vi "Rx Streaming (Four Channels) (Host)(old).vi"() -> ()   [LabVIEW 2021]
doc: "This template is for the Simple NI-USRP Streaming design, a design that shows the basics of streaming data from an NI 294x/295x device. Refer to the block diagram for more information about how to use this template."
uses:
  SubVIs/Start Trigger.ctl
  <vilib>/userdefined/Silver/nirio_resource_slv.ctl
  <vilib>/Utility/error.llb/DialogType.ctl
  <vilib>/measure/maspectr.llb/FFT Power Spectrum and PSD for 1 Chan (CDB).vi
  <vilib>/measure/NI_MAPro.lvlib
panel:
  in  "rx config":T2={"transfer mode"=enum."Finite", "sample rate"=10000000.0, "number of samples"=8192, "start trigger"=enum."Immediate", "daughterboard 0 config"={"rf enable 0"=TRUE, "rf config 0"={"antenna"="RX1", "frequency"=5000000000.0, "gain"=40.0}, "rf enable 1"=TRUE, "rf config 1"={"antenna"="RX2", "frequency"=5000000000.0, "gain"=40.0}, "lo configuration"=enum."Shared"}, "daughterboard 1 config"={"rf enable 2"=TRUE, "rf config 2"={"antenna"="RX1", "frequency"=5000000000.0, "gain"=40.0}, "rf enable 3"=TRUE, "rf config 3"={"antenna"="RX2", "frequency"=5000000000.0, "gain"=40.0}, "lo configuration"=enum."Shared"}} {"daughterboard 1 config"."rf config 3"."gain" format="%#.1f"; "daughterboard 1 config"."rf config 3"."frequency" format="%#.3pHz"; "daughterboard 1 config"."rf config 2"."gain" format="%#.1f"; "daughterboard 1 config"."rf config 2"."frequency" format="%#.3pHz"; "daughterboard 0 config"."rf config 1"."gain" format="%#.1f"; "daughterboard 0 config"."rf config 1"."frequency" format="%#.3pHz"; "daughterboard 0 config"."rf config 0"."gain" format="%#.1f"; "daughterboard 0 config"."rf config 0"."frequency" format="%#.3pHz"; "sample rate" format="%#.3pS/s"}
  out "acquiring":bool caption="Acquiring"
  in  "USRP RIO device":T3="RIO0" caption="USRP RIO Device"
  in  "reference frequency source":string(combo)="Internal" caption="Reference Frequency Source"
  in  "indicator tab":T4(tab)
  out "power spectrum":cluster{"f0":dbl, "df":dbl, "magnitude":dbl[]}[](graph) caption="Power Spectrum"
  out "iq data":waveform(dbl)[](graph) caption="I & Q Data"
  out "rx.coerced config":T5 caption="Coerced Configurations" {"channel 3"."sample rate" format="%#.3pS/s"; "channel 3"."gain" format="%#_1f"; "channel 3"."if2 lo" format="%#.3pHz"; "channel 3"."if1 lo" format="%#.3pHz"; "channel 3"."frequency" format="%#.3pHz"; "channel 2"."sample rate" format="%#.3pS/s"; "channel 2"."gain" format="%#_1f"; "channel 2"."if2 lo" format="%#.3pHz"; "channel 2"."if1 lo" format="%#.3pHz"; "channel 2"."frequency" format="%#.3pHz"; "channel 1"."sample rate" format="%#.3pS/s"; "channel 1"."gain" format="%#_1f"; "channel 1"."if2 lo" format="%#.3pHz"; "channel 1"."if1 lo" format="%#.3pHz"; "channel 1"."frequency" format="%#.3pHz"; "channel 0"."sample rate" format="%#.3pS/s"; "channel 0"."gain" format="%#_1f"; "channel 0"."if2 lo" format="%#.3pHz"; "channel 0"."if1 lo" format="%#.3pHz"; "channel 0"."frequency" format="%#.3pHz"}
  in  "rx.stop":bool
  # "This template shows the basics of streaming data on a USRP-2945/2955 device. Open the Project Documentation folder of the sample project and select Simple NI-USRP Streaming 2945 2955.html for information about using LO sharing with this template."
  # "Simple Rx Streaming"
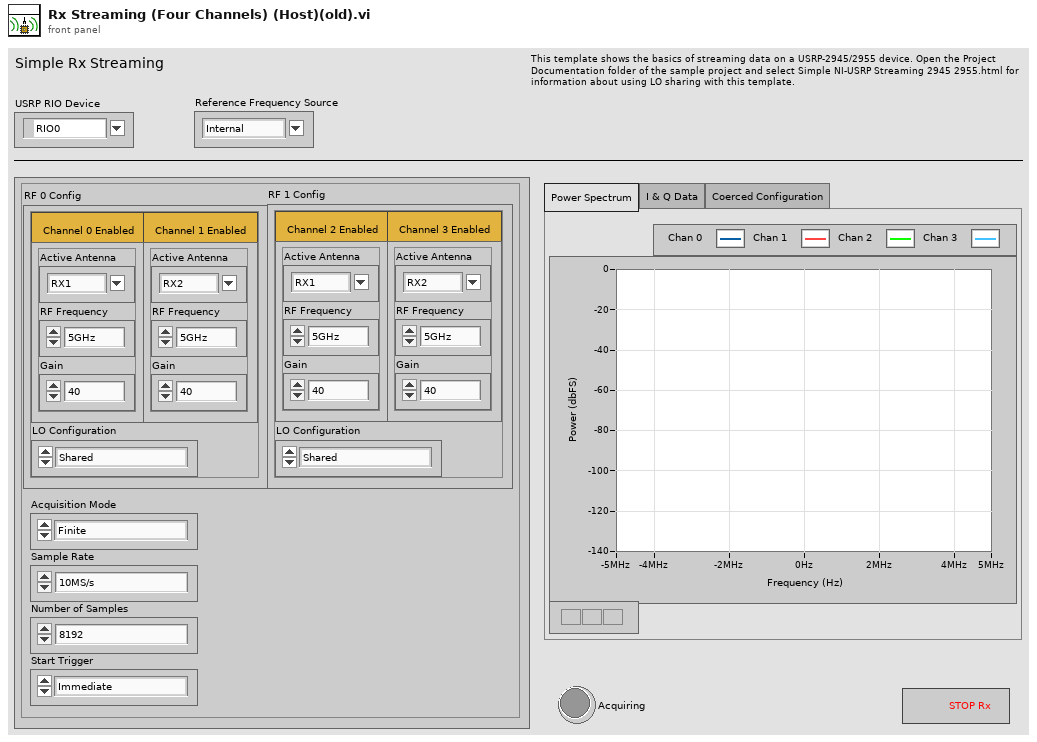
[diagram p1: front panel]
types:
  T1 = typedef "Start Trigger.ctl" = enum8{"Software", "Digital Edge", "Rx Start Trigger", "Tx Start Trigger", "Immediate", "Future Time Event"}
  T2 = cluster{"transfer mode":enum16{"Finite", "Continuous"}, "sample rate":dbl, "number of samples":u32, "start trigger":T1, "daughterboard 0 config":cluster{"rf enable 0":bool, "rf config 0":cluster{"antenna":string, "frequency":dbl, "gain":dbl}, "rf enable 1":bool, "rf config 1":cluster{"antenna":string, "frequency":dbl, "gain":dbl}, "lo configuration":enum16{"Independent", "Import", "Shared and Export", "Reimport", "Shared"}}, "daughterboard 1 config":cluster{"rf enable 2":bool, "rf config 2":cluster{"antenna":string, "frequency":dbl, "gain":dbl}, "rf enable 3":bool, "rf config 3":cluster{"antenna":string, "frequency":dbl, "gain":dbl}, "lo configuration":enum16{"Independent", "Import", "Shared and Export", "Reimport", "Shared"}}}
  T3 = typedef "nirio_resource_slv.ctl" = tag
  T4 = enum32{"Power Spectrum", "I & Q Data", "Coerced Configuration"}
  T5 = cluster{"channel 0":cluster{"frequency":dbl, "if1 lo":dbl, "if2 lo":dbl, "gain":dbl, "sample rate":dbl}[], "channel 1":cluster{"frequency":dbl, "if1 lo":dbl, "if2 lo":dbl, "gain":dbl, "sample rate":dbl}[], "channel 2":cluster{"frequency":dbl, "if1 lo":dbl, "if2 lo":dbl, "gain":dbl, "sample rate":dbl}[], "channel 3":cluster{"frequency":dbl, "if1 lo":dbl, "if2 lo":dbl, "gain":dbl, "sample rate":dbl}[], "device id":i32}
  T6 = typedef "DialogType.ctl" = u16
  T7 = typedef "Rx Channels.ctl" = cluster{"rx config":cluster{"channel configuration":cluster{"channel enable":bool, "channel configuration":cluster{"antenna":string, "frequency":dbl, "lo frequency":dbl, "level":dbl}}[], "transfer mode":enum16{"Finite", "Continuous"}, "sample rate":dbl, "number of samples":u32, "start trigger":T1}, "reference frequency source":string, "rx.data sink":enum16{"SFP Port 0", "SFP Port 1", "Host"}, "rx.enabled channels":string[], "vertical range":dbl[], "rx.coerced configurations":cluster{"coerced frequencies":dbl[], "coerced lo frequencies":dbl[], "coerced levels":dbl[], "coerced sample rates":dbl[]}}
  T8 = typedef "niUsrpRio Config v1 Host.lvlib/niUsrpRio Session.ctl" = cluster{"FPGA Interface":refnum<k20>, "RIO Interface Number":u32, "Data Clock Rate":u32, "FPGA Data Clock Rate":u32, "Global Settings Register Bus":T9, "Radio 0 Settings Register Bus":T9, "Radio 1 Settings Register Bus":T9, "Radio Settings Bus Semaphore":T10, "DB Queues":T11[], "Characterization Data Valid?":bool, "EEPROM Header":T12, "Device Data Header":T13, "EEPROM Characterization Header":T14, "Characterization Data":T15[], "FPGA Current Version":u32, "FPGA Oldest Compatible Version":u32, "Fixed Logic Current Version":u32, "Fixed Logic Oldest Compatible Version":u32, "FPGA Radio Settings Bus Current Version":u32, "FPGA Radio Settings Bus Oldest Compatible Version":u32, "FPGA Board Config Current Version":u32, "FPGA Board Config Oldest Compatible Version":u32, "Daughterboard Clock Rate":u32, "daughterboard configuration session handles":u64[]}
  T9 = typedef "niInstr Register Bus v0 Host.lvlib/Register Bus Session.ctl" = refnum<queue>
  T10 = typedef "Semaphore RefNum" = refnum<k1>
  T11 = typedef "niUsrpRio Config v1 Host.lvlib/DB Queue Reference.ctl" = refnum<queue>
  T12 = typedef "niUsrpRio Config v1 Host.lvlib/EEPROM Header.ctl" = cluster{"Checksum":u32, "Product Code":u16, "Hardware Current Version":u16, "Hardware Oldest Compatible Version":u16, "EEPROM Map Current Version":u16, "EEPROM Map Oldest Compatible Version":u16, "User Password":string, "Pointer to Factory Header":u32, "Pointer to User Header":u32, "Recommended Interval":u16, "Number of Reserved Bytes":i32, "Number of Daughterboards":u8, "Daughterboard IDs":u16[], "Daughterboard Serial Numbers":string[]}
  T13 = typedef "niUsrpRio Config v1 Host.lvlib/EEPROM Device Data Header.ctl" = cluster{"Checksum":u32, "Number of Channels":u8, "Number of Gain Settings":u16[], "Pointer to Characterization Data":u32[], "Number of Reserved Bytes":i32, "Number of Frequencies":u16[]}
  T14 = typedef "niUsrpRio Config v1 Host.lvlib/EEPROM Characterization Header.ctl" = cluster{"Checksum":u32, "Date":timestamp, "Temperature":sgl, "Misc. Info":string, "Pointer to Device Data Header":u32, "Number of Reserved Bytes":i32}
  T15 = typedef "niUsrpRio Config v1 Host.lvlib/Characterization Data.ctl" = cluster{"Gains[dB]":dbl[], "Frequencies [Hz]":dbl[], "IQ Imbalance Table":T16[], "Measured Gains[dB]":dbl[][]}
  T16 = typedef "niUsrpRio Config v1 Host.lvlib/IQ Imbalance.ctl" = cluster{"Gain Imbalance [linear]":dbl, "Phase Imbalance [radians]":dbl, "Offset":cdb}
  T17 = cluster{"coerced frequencies":dbl[], "coerced if1 frequencies":dbl[], "coerced if2 frequencies":dbl[], "coerced gain":dbl[], "coerced sample rates":dbl[]}
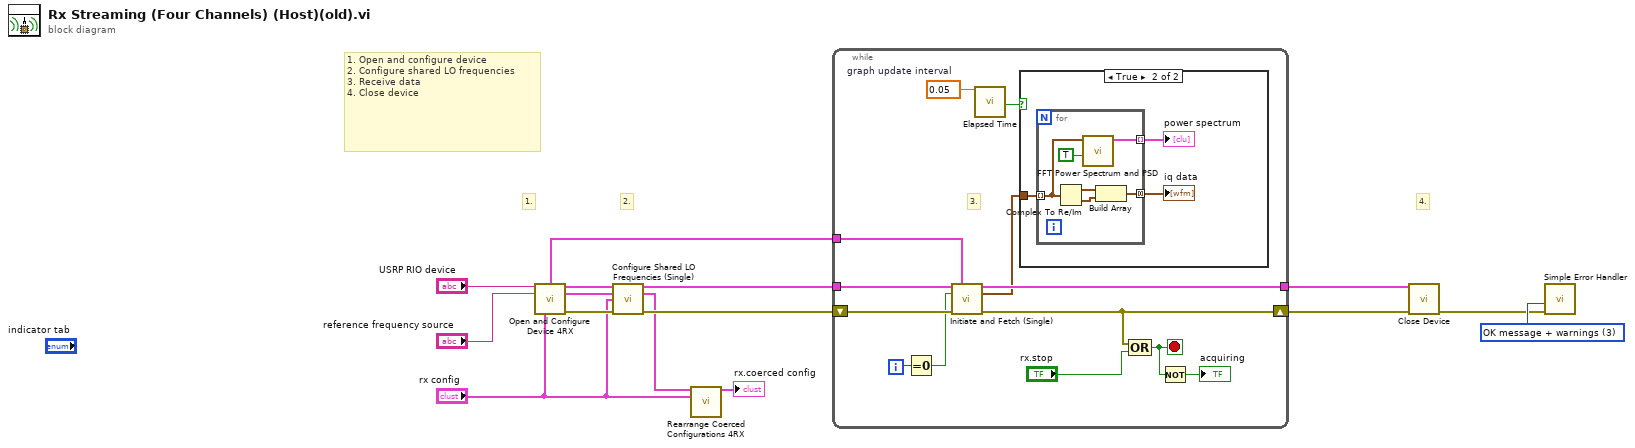
[diagram p0: block diagram]
diagram:
  w15 = T6 3 items=["no dialog", "OK message", "continue or stop message", "OK message + warnings", "continue/stop + warnings"] ("type of dialog (OK msg:1)")
  # "2."
  # "4."
  # "1. Open and configure device\n2. Configure shared LO frequencies\n3. Receive data\n4. Close device"
  # "1."
  n1 = call "Open and Configure Device 4RX.vi"("USRP RIO Device"="USRP RIO device", "reference frequency source"="reference frequency source", "rx config"="rx config") -> ("rx channels"=w9:T7, "niUsrpRio Session (out)"=w7:T8, "rx.coerced configurations"=w3:T17, "error out"=w4:errorcluster)  [unwired: 9 in]
  n2 = call "Configure Shared LO Frequencies (Single).vi"("niUsrpRio Session"=w7, "rx.coerced config"=w3, "rx config"="rx config", "error in"=w4) -> ("niUsrpRio Session (out)"=w6:T8, "rx.coerced config out"=w1:T17, "error out"=w5:errorcluster)  [unwired: 9 in]
  n3 = call "Rearrange Coerced Configurations 4RX.vi"("rx.coerced configurations"=w1, "rx config"="rx config") -> ("coerced configurations"=→"rx.coerced config":T5)  [unwired: 13 in]
  n4 = while {
    tunnel: w6 -> [w26]
    tunnel: [w23] -> w10
    tunnel: w9 -> [w20]
    shift-right: [w24] -> w11
    shift-left: w5 -> [w27]
    i -> [w25]
    stop <- w21 stop-if-true
    w18 = 0.05  # graph update interval
    # "3."
    # "Acquire and Fetch a waveform"
    n5 = Equal To 0?(x=w25) -> (x = 0?=w16:bool)
    n6 = call "Initiate and Fetch (Single).vi"("niUsrpRio Session"=w26, "rx channels"=w20, "first iteration"=w16, "error in"=w27) -> ("niUsrpRio Session (out)"=w23:T8, "complex baseband data"=w17:waveform(cdb)[], "error out"=w24:errorcluster)  [unwired: 9 in]
    n7 = call "Elapsed Time"("Time Target (s)"=w18) -> ("Time has Elapsed"=w19:bool)  [unwired: 11 in, 7 out]
    n8 = case shown="True" w19 {
      tunnel: w17 -> [_ w31]
      frame False {
      }
      frame True {
        n9 = for {
          tunnel: [w35] -> w30 mode=concatenating
          tunnel: [w33] -> w29 mode=indexing
          tunnel: w31 -> [w34] mode=indexing
          n10 = Complex To Re/Im(x + iy=w34) -> (x=w37:waveform(dbl), y=w36:waveform(dbl))
          n11 = call-poly <vilib>:"FFT Power Spectrum and PSD.vi"("dB On (F)"=TRUE, "time signal"=w34) -> ("Power Spectrum / PSD"=w33:cluster{"f0":dbl, "df":dbl, "magnitude":dbl[]})  [unwired: 6 in, 3 out]
          n12 = Build Array(w37, w36) -> (w35:waveform(dbl)[])
        }
        "power spectrum" <- w29
        "iq data" <- w30
      }
    }
    n13 = Compound Arithmetic op=OR(w24, "rx.stop") -> (w21:bool)
    n14 = Not(x=w21) -> (.not. x?=→"acquiring":bool)
  }
  n15 = call "Close Device.vi"("niUsrpRio Session"=w10, "error in"=w11) -> ("error out"=w14:errorcluster)  [unwired: 13 in]
  n16 = call <vilib>:"Simple Error Handler.vi"("type of dialog (OK msg:1)"=w15, "error in (no error)"=w14) -> ()  [unwired: 3 in, 5 out]
